vi "Tray_SetTrayColorData.vi"(6 "Color":u32, 8 "error in (no error)":errorcluster, 9 "Index":cluster{"X":i32, "Y":i32}, 10 "Data":string, 11 "TrayRef":refnum<vi>) -> (0 "error out":errorcluster)   [LabVIEW 2019]
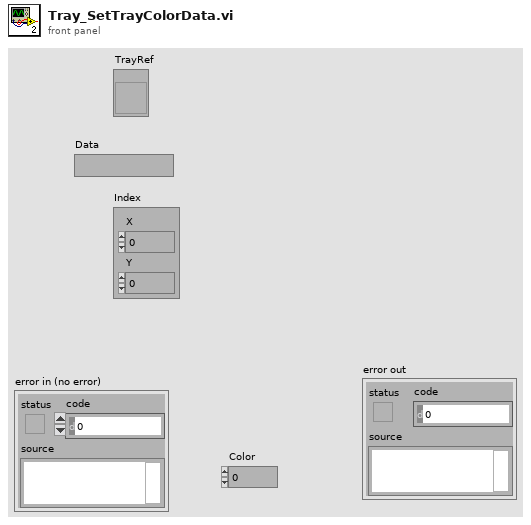
[diagram p1: front panel]
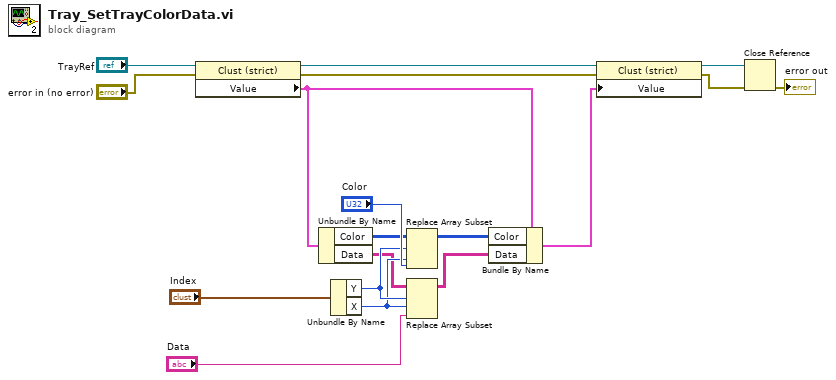
[diagram p0: block diagram]
diagram:
  n1 = property class="Clust (strict)"(reference="TrayRef", error in="error in (no error)") -> (reference out=w16:refnum<vi>, error out=w3:errorcluster, "Value"=w15:cluster{"Color":u32[][], "Data":string[][]})
  n2 = Unbundle By Name(w15) -> ("Color"=w11:u32[][], "Data"=w6:string[][])
  n3 = Unbundle By Name("Index") -> ("Y"=w8:i32, "X"=w7:i32)
  n4 = Replace Array Subset(array=w11, new element="Color", index (row)=w8, index (col)=w7) -> (w13:u32[][])
  n5 = Replace Array Subset(array=w6, new element="Data", index (row)=w8, index (col)=w7) -> (w18:string[][])
  n6 = Bundle By Name(cluster=w15, "Color"=w13, "Data"=w18) -> (w17:cluster{"Color":u32[][], "Data":string[][]})
  n7 = property class="Clust (strict)"(reference=w16, error in=w3, "Value"=w17) -> (reference out=w5:refnum<vi>, error out=w2:errorcluster)
  n8 = Close Reference(reference=w5, error in (no error)=w2) -> (error out=→"error out":errorcluster)
